vi "example.vi"() -> ()   [LabVIEW 2021]
uses:
  Servo drive module.lvlib
  ctl/Servo over status.ctl
  ctl/Servo status variable.ctl
  ctl/Servo status constants.ctl
panel:
  out "Status out":T1
  in  "MAG config file path":path=path "Y:/Instrument/Software/UI/SystemData/testconfig.ini"
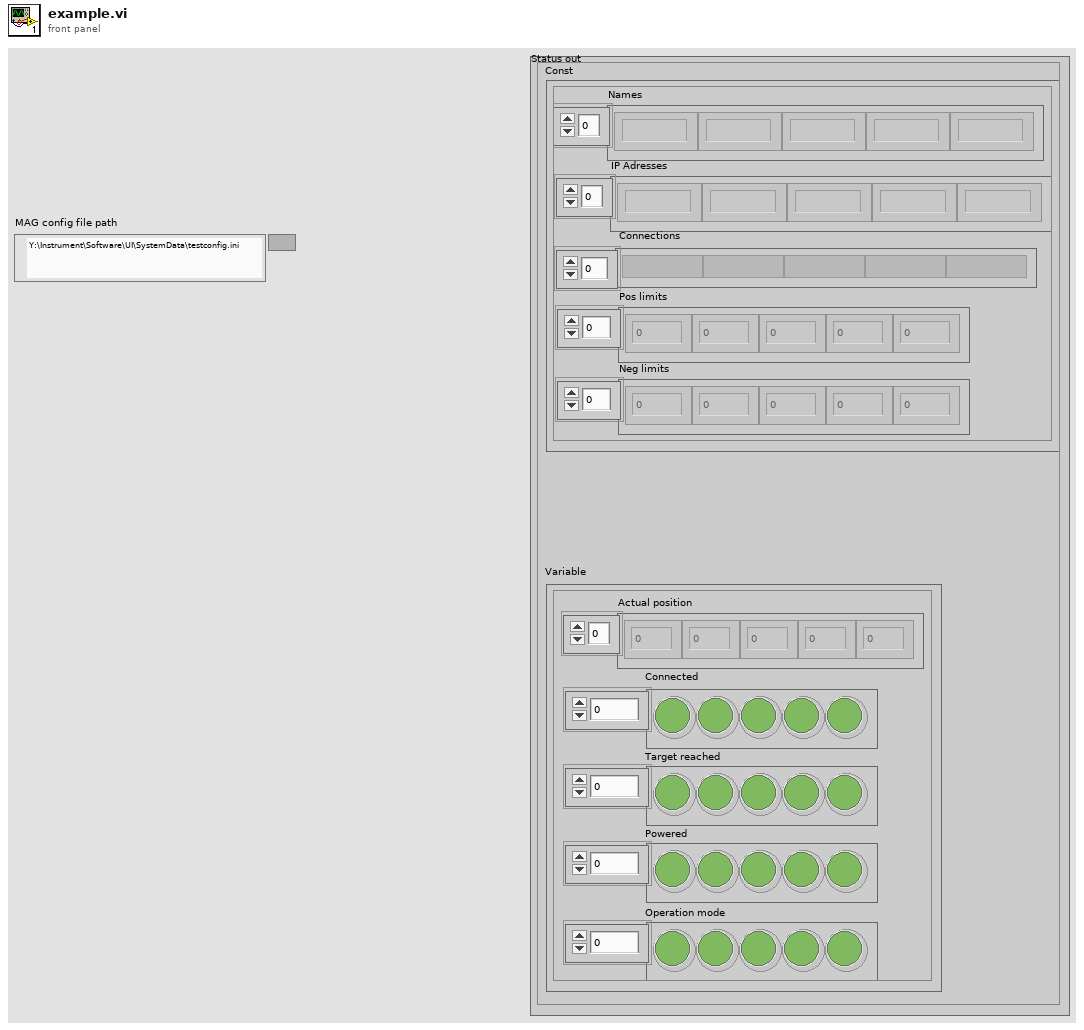
[diagram p1: front panel]
types:
  T1 = typedef "Servo over status.ctl" = cluster{"Variable":T2, "Const":T3}
  T2 = typedef "Servo status variable.ctl" = cluster{"Connected":bool[], "Target reached":bool[], "Powered":bool[], "Actual position":dbl[], "Operation mode":bool[]}
  T3 = typedef "Servo status constants.ctl" = cluster{"IP Adresses":string[], "Names":string[], "Connections":variant[], "Pos limits":dbl[], "Neg limits":dbl[]}
  T4 = typedef "Servo drive module.lvlib/Servo state.ctl" = cluster{"Servo variables":T5, "Servo constants":T6, "Connection":variant}
  T5 = typedef "Servo drive module.lvlib/Servo variables.ctl" = cluster{"Terget reached":bool, "Connected":bool, "Power ON":bool, "Operation mode":bool, "Actual position":dbl, "Target position":dbl}
  T6 = typedef "Servo drive module.lvlib/Servo constants.ctl" = cluster{"Name":T7, "Pos position limit [mm]":dbl, "Neg position limit [mm]":dbl, "Pos velocity limit":dbl, "Neg velocity limit":dbl, "Acceleration limit":dbl}
  T7 = typedef "Servo drive module.lvlib/Axis names.ctl" = enum16{"Unknown", "AxisX", "AxisY", "AxisZ_left", "AxisZ_middle", "AxisZ_right"}
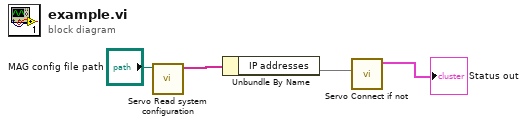
[diagram p0: block diagram]
diagram:
  n1 = call "Servo Read system configuration.vi"("MAG config file path"="MAG config file path") -> ("IP addresses"=w3:string[])  [unwired: 8 in, 2 out]
  n2 = Unbundle By Name(w3) -> ("IP addresses"=w2)
  n3 = call "Servo Connect if not.vi"("IP addresses"=w2) -> ("Servo statuses"=→"Status out":T4[])  [unwired: 9 in, 1 out]
